vi "Write DUT Info.vi"(8 "error in (no error)":errorcluster, 10 "DUT Info":T1, 11 "Results List in":refnum<class "Results List.lvclass">) -> (0 "error out":errorcluster, 3 "Results List out":refnum<class "Results List.lvclass">)   [LabVIEW 2015, in "Results List.lvclass"]
uses:
  Results List.lvclass
  DUT Information.ctl
  Results List.lvclass/Results List.ctl
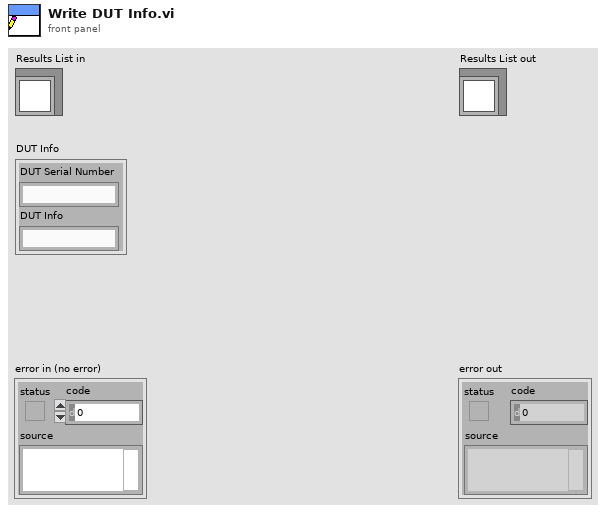
[diagram p1: front panel]
types:
  T1 = typedef "Results List.lvclass/DUT Information.ctl" = cluster{"DUT Serial Number":string, "DUT Info":string}
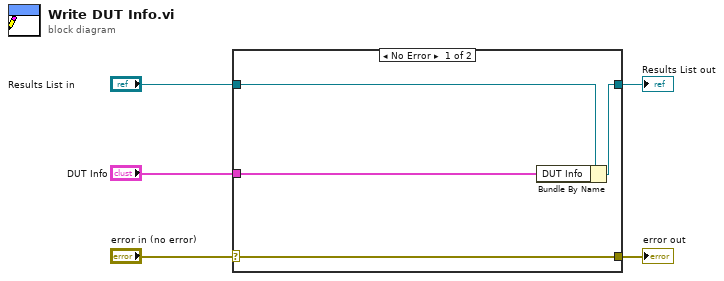
[diagram p0: block diagram]
diagram:
  n1 = case shown="No Error" "error in (no error)" {
    selector: "error in (no error)" -> [w9 w10]
    tunnel: [w9 w10] -> w4
    tunnel: [w7 w11] -> w2
    tunnel: "Results List in" -> [w8 w11]
    tunnel: "DUT Info" -> [w6 _]
    frame No Error {
      n2 = Bundle By Name(cluster=w8, "DUT Info"=w6) -> (w7:refnum<class "Results List.lvclass">)
    }
    frame Error {
    }
  }
  "error out" <- w4
  "Results List out" <- w2
